vi "Set NI-SWITCH Topology.vi"(8 "error in":errorcluster, 10 "topology":string, 11 "ni-switch custom device in":T1 format="%.0x") -> (0 "error out":errorcluster, 3 "ni-switch custom device out":T1 format="%.0x")   [LabVIEW 2017, in "NI-SWITCH Scripting.lvlib"]
doc: "Sets the topology for the SLSC Switch custom device."
uses:
  NI-SWITCH Scripting.lvlib
  <vilib>/NI Veristand/Custom Device API/Custom Device Item Ref.ctl
  <vilib>/NI VeriStand/Custom Device API/Custom Device API.lvlib
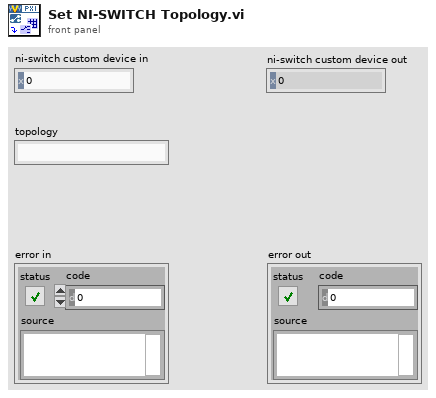
[diagram p1: front panel]
types:
  T1 = typedef "Custom Device API.lvlib/Custom Device Item Ref.ctl" = u64
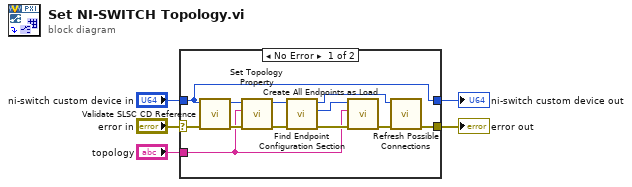
[diagram p0: block diagram]
diagram:
  n1 = case shown="No Error" "error in" {
    selector: "error in" -> [w9 w19]
    tunnel: "topology" -> [w6 _]
    tunnel: [w13 w19] -> w5
    tunnel: "ni-switch custom device in" -> [w10 w18]
    tunnel: [w10 w18] -> w2
    frame No Error {
      n2 = call "Validate SLSC CD Reference.vi"("error in"=w9, "ni-switch custom device in"=w10) -> ("error out"=w11:errorcluster, "ni-switch custom device out"=w12:T1)  [unwired: 8 in]
      n3 = call "Set Topology Property.vi"("error in"=w11, "topology"=w6, "ni-switch custom device in"=w12) -> ("error out"=w7:errorcluster, "ni-switch custom device out"=w8:T1)  [unwired: 7 in]
      n4 = call "Find Endpoint Configuration Section.vi"("error in"=w7, "ni-switch custom device in"=w8) -> ("error out"=w15:errorcluster, "endpoint configuration"=w16:T1, "ni-switch custom device out"=w17:T1)  [unwired: 7 in]
      n5 = call "Create All Endpoints as Load.vi"("error in"=w15, "topology"=w6, "endpoint configuration in"=w16) -> ("error out"=w14:errorcluster)  [unwired: 7 in, 1 out]
      n6 = call "Refresh Possible Connections.vi"("error in"=w14, "ni-switch custom device in"=w17) -> ("error out"=w13:errorcluster)  [unwired: 8 in, 1 out]
    }
    frame Error {
    }
  }
  "error out" <- w5
  "ni-switch custom device out" <- w2
